vi "Wavelength PEM and Digikröm.vi"(8 "error in (no error)":errorcluster, 10 "Spectrometer Digikröm.lvclass":refnum<class "Spectrometer Digikröm.lvclass">, 11 "Wavelength PEM and Digikröm in":refnum<class "Wavelength PEM and Digikröm.lvclass">) -> (0 "error out":errorcluster, 3 "Wavelength PEM and Digikröm out":refnum<class "Wavelength PEM and Digikröm.lvclass">)   [LabVIEW 2017, in "Wavelength PEM and Digikröm.lvclass"]
uses:
  C:/LabVIEW-programs/Scanners/Scanner/Scanner.lvclass
  C:/LabVIEW-programs/Instruments/Utility Classes/Scannable/Scannable.lvclass
  Global/GPIB Numbers.vi
  Scanner/Scanner.lvclass
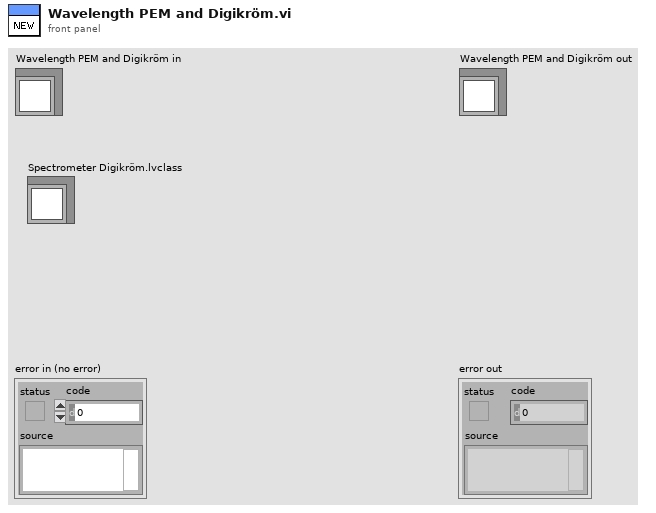
[diagram p1: front panel]
types:
  T1 = typedef "GPIB Type Def.ctl" = cluster{"Name":string, "bus":dbl, "GPIB":dbl, "GPIB as string":string, "byte":i32, "VISA Resource Name":refnum<visa-resource-name>}
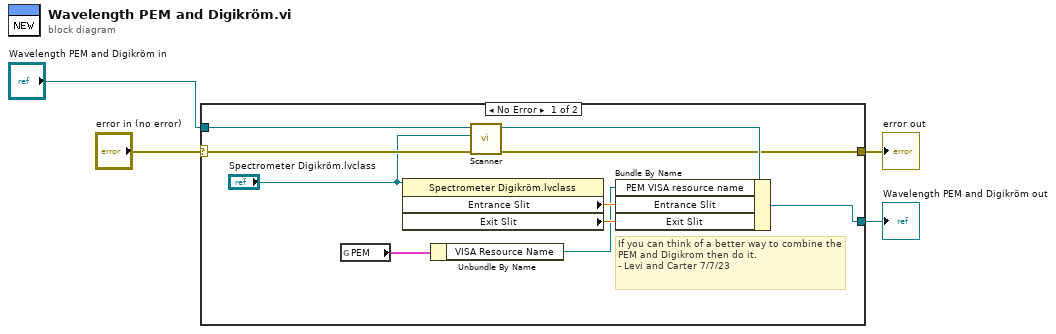
[diagram p0: block diagram]
diagram:
  n1 = case shown="No Error" "error in (no error)" {
    selector: "error in (no error)" -> [w14 w16]
    tunnel: [w11 w16] -> w2
    tunnel: [w7 w15] -> w1
    tunnel: "Wavelength PEM and Digikröm in" -> [w12 w15]
    frame No Error {
      # "If you can think of a better way to combine the PEM and Digikrom then do it.\n- Levi and Carter 7/7/23"
      n2 = global read "GPIB Numbers.vi" "PEM"() -> (w6:T1)
      n3 = property class="Spectrometer Digikröm.lvclass"(reference="Spectrometer Digikröm.lvclass") -> ("Entrance Slit"=w10:dbl[unit], "Exit Slit"=w9:dbl[unit])  [unwired: 1 in, 2 out]
      n4 = Unbundle By Name(w6) -> ("VISA Resource Name"=w5:refnum<visa-resource-name>)
      n5 = call "Scanner.vi"("error in (no error)"=w14, "Scannable"="Spectrometer Digikröm.lvclass", "Scanner.lvclass in"=w12) -> ("error out"=w11:errorcluster, "Scanner.lvclass out"=w13:refnum<class "Wavelength PEM and Digikröm.lvclass">)  [unwired: 1 in, 6 out]
      n6 = Bundle By Name(cluster=w13, "PEM VISA resource name"=w5, "Entrance Slit"=w10, "Exit Slit"=w9) -> (w7:refnum<class "Wavelength PEM and Digikröm.lvclass">)
    }
    frame Error {
    }
  }
  "error out" <- w2
  "Wavelength PEM and Digikröm out" <- w1
